vi "Draw Overlays.vi"(8 "error in (no error)":errorcluster, 11 "Rectangle in":refnum<class "Layered Shape.lvclass">) -> (0 "error out":errorcluster, 2 "Overlays":string[](array[string]), 3 "Rectangle out":refnum<class "Layered Shape.lvclass">)   [LabVIEW 2015, in "LV Image Editor Framework.lvlib" / "Layered Shape.lvclass"]
uses:
  Layered Shape.lvclass
  Layered Shape.lvclass/Layered Shape.ctl
  Shape/Shape.lvclass
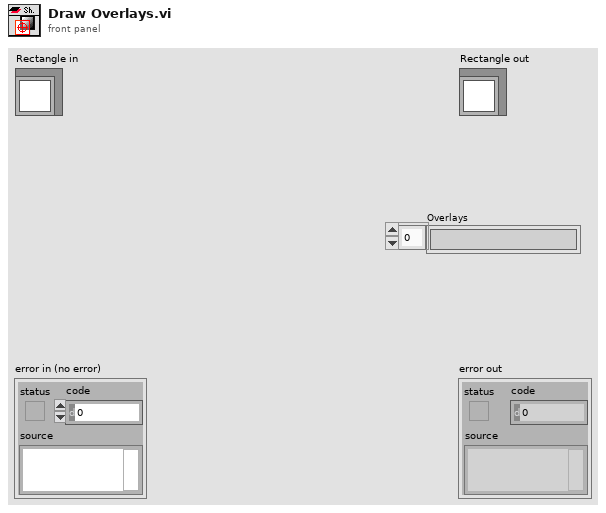
[diagram p1: front panel]
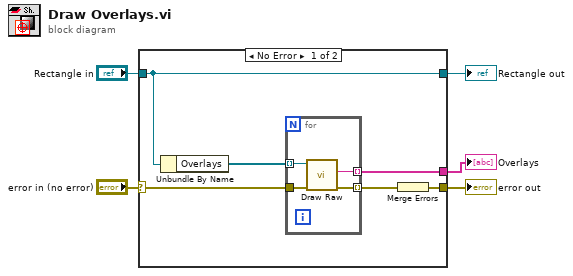
[diagram p0: block diagram]
diagram:
  n1 = case shown="No Error" "error in (no error)" {
    selector: "error in (no error)" -> [w10 w17]
    tunnel: [w8 w17] -> w4
    tunnel: [w11 w16] -> w2
    tunnel: "Rectangle in" -> [w11 w16]
    tunnel: [w7 _] -> w1
    frame No Error {
      n2 = Unbundle By Name(w11) -> ("Overlays"=w6:refnum<class "Shape.lvclass">[])
      n3 = for {
        tunnel: w10 -> [w15]
        tunnel: [w14] -> w7 mode=indexing
        tunnel: [w13] -> w9 mode=indexing
        tunnel: w6 -> [w12] mode=indexing
        n4 = call "Draw Raw.vi"("error in (no error)"=w15, "Shape in"=w12) -> ("error out"=w13:errorcluster, "Raw"=w14:string)  [unwired: 7 in, 1 out]
      }
      n5 = Merge Errors(w9) -> (w8:errorcluster)
    }
    frame Error {
    }
  }
  "error out" <- w4
  "Rectangle out" <- w2
  "Overlays" <- w1
